vi "RPMtoSpeed.vi"(2 "Speed":dbl, 3 "Measured RPM":dbl, 4 "Desired RPM":dbl) -> (0 "New Speed":dbl, 1 "Update?":bool)   [LabVIEW 2017]
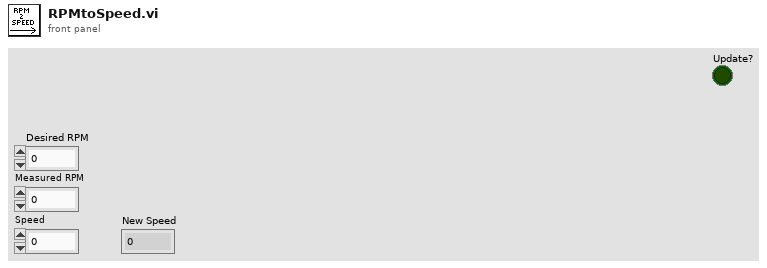
[diagram p1: front panel]
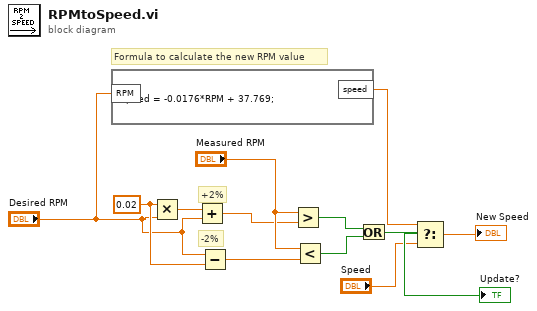
[diagram p0: block diagram]
diagram:
  w11 = 0.02 ("x")
  # "Formula to calculate the new RPM value"
  # "-2%"
  # "+2%"
  n1 = formula code="speed = -0.0176*RPM + 37.769;"("RPM"="Desired RPM") -> ("speed"=w1:dbl)
  n2 = Multiply(x=w11, y="Desired RPM") -> (x*y=w12:dbl)
  n3 = Add(x=w12, y="Desired RPM") -> (x+y=w9:dbl)
  n4 = Subtract(x="Desired RPM", y=w11) -> (x-y=w8:dbl)
  n5 = Greater?(x="Measured RPM", y=w9) -> (0:w7:bool)
  n6 = Less?(x="Measured RPM", y=w8) -> (x < y?=w6:bool)
  n7 = Or(x=w7, y=w6) -> (x .or. y?=w5:bool)
  "Update?" <- w5
  n8 = Select(t=w1, s=w5, f="Speed") -> (s? t:f=→"New Speed":dbl)
